vi "Reference Cluster MsgPack Example.vi"() -> ()   [LabVIEW 2015, in "MsgPack.lvlib"]
uses:
  MsgPack.lvlib
  Complex Cluster.ctl
  Simple Cluster.ctl
panel:
  out "Complex MsgPack Data":string
  out "Received Simple":T1 {"Single" format="%#.19f"}
  out "Simple":T1 {"Single" format="%#.19f"}
  out "Received Complex":T2 {"ArrayOfClusters"."Single" format="%#.19f"; "NestedCluster"."Single" format="%#.19f"}
  out "Complex Decode Error":errorcluster
  out "Simple Decode Error":errorcluster
  in  "Flag":bool=TRUE
  out "Simple MsgPack Data":string
  in  "Array Size":i32=5
  out "Complex":T2 {"ArrayOfClusters"."Single" format="%#.19f"; "NestedCluster"."Single" format="%#.19f"}
  # "This Example VI shows a way to send a complex Cluster over MsgPack.  This is an extenstion to the \"Simple Cluster MsgPack Example.vi\" and \"Complex Cluster MsgPack Example.vi\"\n\nThis examples uses Cluster References to do the tedious work of loading all the cluster keys with the appropiate values.\n\n\n1 - The Time is autopopulated with the current timestamp.  This shows how the MsgPack EXT datatype can be used for sending custom data types.  A Timestamp (EXT type = -1) is defined by the MsgPack Standard and is included as an example.\n2 - Try setting different values for \"FLAG\" and \"Array Size\".\n\nNote: The real magic works in the \"variantClusterByRef.vi\" where the cluster reference is examined and the appropiate key-value relationships are evaulated and updated."
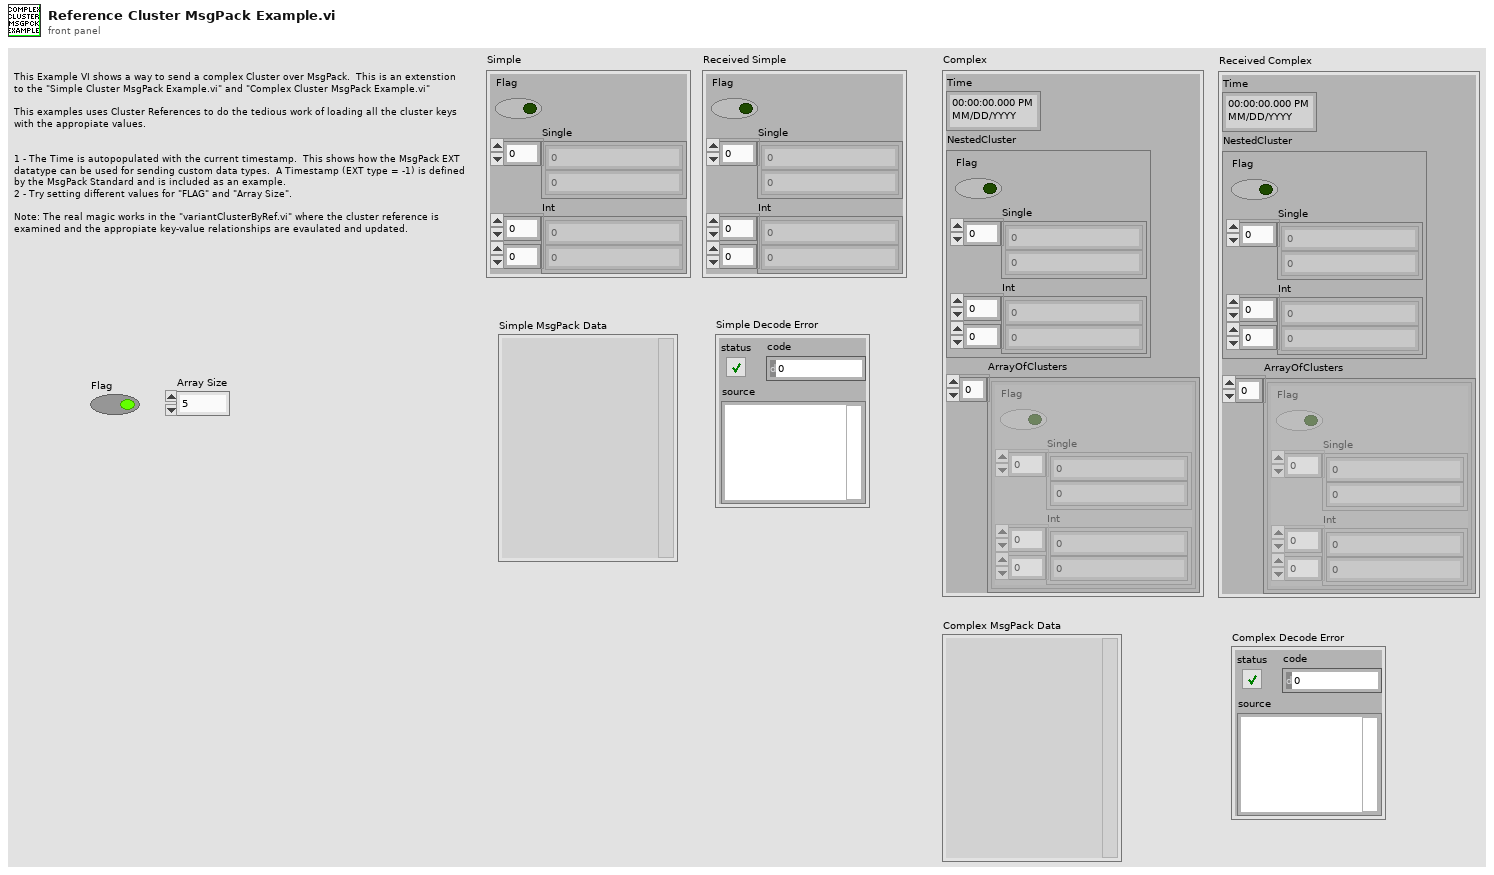
[diagram p1: front panel]
types:
  T1 = typedef "MsgPack.lvlib/Simple Cluster.ctl" = cluster{"Flag":bool, "Single":sgl[], "Int":i32[][]}
  T2 = typedef "MsgPack.lvlib/Complex Cluster.ctl" = cluster{"Time":timestamp, "NestedCluster":T1, "ArrayOfClusters":T1[]}
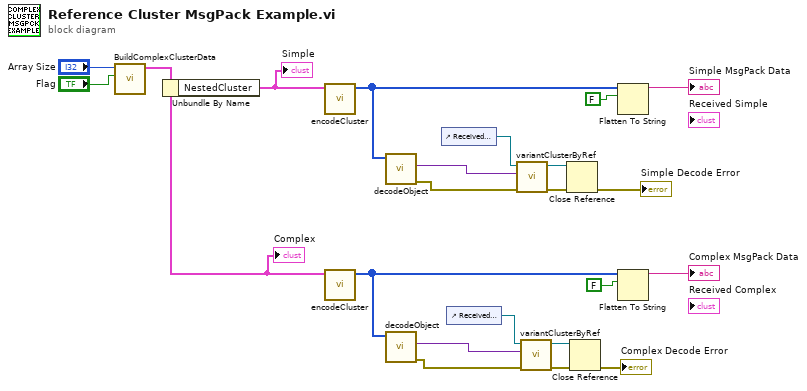
[diagram p0: block diagram]
diagram:
  n1 = call "BuildComplexClusterData.vi"("Flag"="Flag", "Array Size"="Array Size") -> ("Packet"=w12:T2)  [unwired: 9 in]
  "Complex" <- w12
  n2 = Unbundle By Name(w12) -> ("NestedCluster"=w11:T1)
  "Simple" <- w11
  n3 = call "encodeCluster.vi"("Variant"=w11) -> ("MessagePack"=w20:u8[])  [unwired: 9 in, 1 out]
  n4 = call "encodeCluster.vi"("Variant"=w12) -> ("MessagePack"=w16:u8[])  [unwired: 9 in, 1 out]
  n5 = call "decodeObject.vi"("ByteArray"=w20) -> ("error out"=w19:errorcluster, "Variant"=w7:variant)  [unwired: 7 in, 2 out]
  n6 = call "decodeObject.vi"("ByteArray"=w16) -> ("error out"=w15:errorcluster, "Variant"=w9:variant)  [unwired: 7 in, 2 out]
  n7 = control-ref of="Received Simple"() -> (w8:refnum<vi>)
  n8 = control-ref of="Received Complex"() -> (w10:refnum<vi>)
  n9 = call "variantClusterByRef.vi"("error in (no error)"=w19, "MsgPack Variant"=w7, "Cluster Reference"=w8) -> ("error out"=w5:errorcluster, "Cluster Reference (dup)"=w6:refnum<vi>)  [unwired: 7 in]
  n10 = call "variantClusterByRef.vi"("error in (no error)"=w15, "MsgPack Variant"=w9, "Cluster Reference"=w10) -> ("error out"=w3:errorcluster, "Cluster Reference (dup)"=w2:refnum<vi>)  [unwired: 7 in]
  n11 = Close Reference(reference=w6, error in (no error)=w5) -> (error out=→"Simple Decode Error":errorcluster)
  n12 = Close Reference(reference=w2, error in (no error)=w3) -> (error out=→"Complex Decode Error":errorcluster)
  n13 = Flatten To String(anything=w20, prepend array or string size? (T)=FALSE) -> (data string=→"Simple MsgPack Data":string)  [unwired: 2 in, 2 out]
  n14 = Flatten To String(anything=w16, prepend array or string size? (T)=FALSE) -> (data string=→"Complex MsgPack Data":string)  [unwired: 2 in, 2 out]
